vi "Test 2.vi"() -> ()   [LabVIEW 2015]
uses:
  Control test 1.ctl
  <vilib>/Waveform/WDTOps.llb/WDT Append Waveforms DBL.vi
panel:
  in  "maximumTolerance":dbl
  in  "minimumTolerance":dbl
  in  "targetPressure":dbl
  out "target_pr":dbl
  out "current pr":dbl
  out "data":T1
  in  "stop (F)":bool
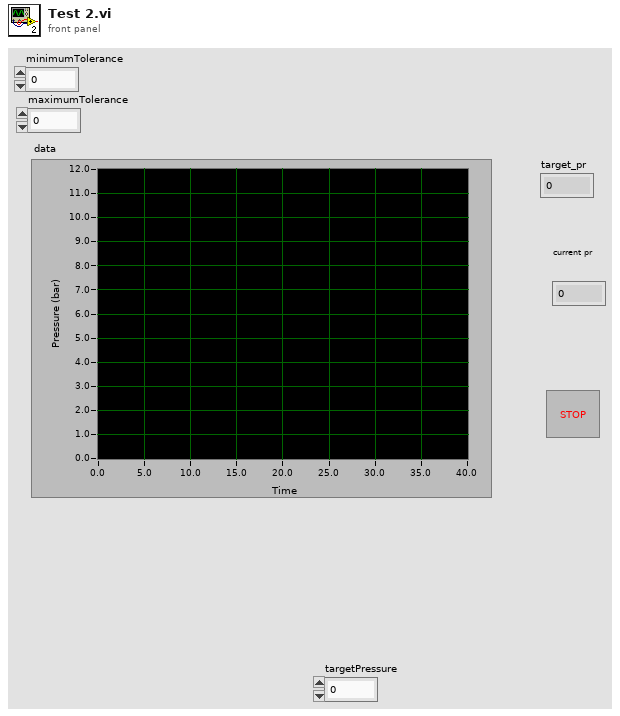
[diagram p1: front panel]
types:
  T1 = typedef "Control test 1.ctl" = dynamicdata
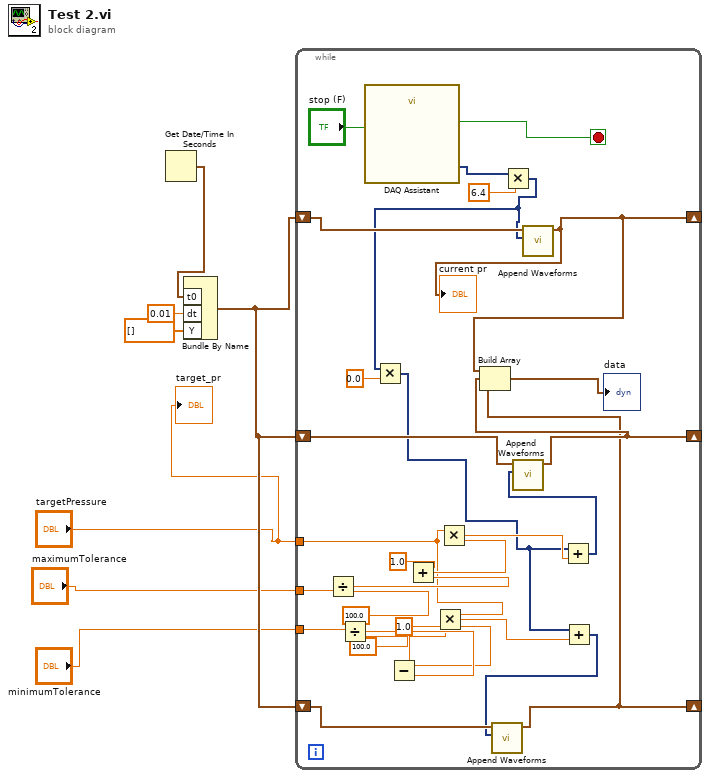
[diagram p0: block diagram]
diagram:
  n1 = Get Date/Time In Seconds() -> (seconds since 1Jan1904=w5:timestamp)
  n2 = Bundle By Name("t0"=w5, "dt"=0.01, "Y"=dbl[] []) -> (w4:waveform(dbl))  [unwired: 1 in]
  n3 = while {
    shift-right: [w31] -> _
    shift-left: w4 -> [w32]
    shift-right: [w28] -> _
    shift-left: w4 -> [w29]
    tunnel: "maximumTolerance" -> [w27]
    tunnel: "minimumTolerance" -> [w25]
    tunnel: "targetPressure" -> [w17]
    shift-right: [w11] -> _
    shift-left: w4 -> [w12]
    stop <- w35 stop-if-true
    n4 = Divide(x=w27, y=100.0) -> (x/y=w22:dbl)
    n5 = Divide(x=w25, y=100.0) -> (x/y=w21:dbl)
    n6 = call "DAQ Assistant"("stop (F)"="stop (F)") -> ("data"=w33:dynamicdata, "stopped"=w35:bool)  [unwired: 15 in, 2 out]
    n7 = Subtract(x=1.0, y=w21) -> (x-y=w19:dbl)
    n8 = Add(x=1.0, y=w22) -> (x+y=w18:dbl)
    n9 = Multiply(x=w17, y=w19) -> (x*y=w9:dbl)
    n10 = Multiply(x=w17, y=w18) -> (x*y=w14:dbl)
    n11 = Multiply(x=w33, y=6.4) -> (x*y=w16:dynamicdata)
    n12 = Multiply(x=w16, y=0.0) -> (x*y=w10:dynamicdata)
    n13 = call-poly <vilib>:"Append Waveforms.vi"("waveform B"=w16, "waveform A"=w32) -> ("waveform out"=w31:waveform(dbl))  [unwired: 8 in, 1 out]
    "current pr" <- w31
    n14 = Add(x=w10, y=w14) -> (x+y=w13:dynamicdata)
    n15 = call-poly <vilib>:"Append Waveforms.vi"("waveform B"=w13, "waveform A"=w29) -> ("waveform out"=w28:waveform(dbl))  [unwired: 8 in, 1 out]
    n16 = Add(x=w10, y=w9) -> (x+y=w8:dynamicdata)
    n17 = call-poly <vilib>:"Append Waveforms.vi"("waveform B"=w8, "waveform A"=w12) -> ("waveform out"=w11:waveform(dbl))  [unwired: 8 in, 1 out]
    n18 = Build Array(w31, w28, w11) -> (→"data":waveform(dbl)[])
  }
  "target_pr" <- "targetPressure"
